vi "Create Table.vi"(8 "error in (no error)":errorcluster, 9 "New Table Name":string, 10 "Table Paths":string[](array[string]), 11 "Data.PGSQL":refnum<class "LV-Data.PGSQL.lvclass">) -> (0 "error out":errorcluster, 3 "Data.PGSQL out":refnum<class "LV-Data.PGSQL.lvclass">)   [LabVIEW 2019, in "LV-Data.PGSQL.lvclass"]
uses:
  LV-Data.PGSQL.lvclass
panel:
  in  "OK":bool
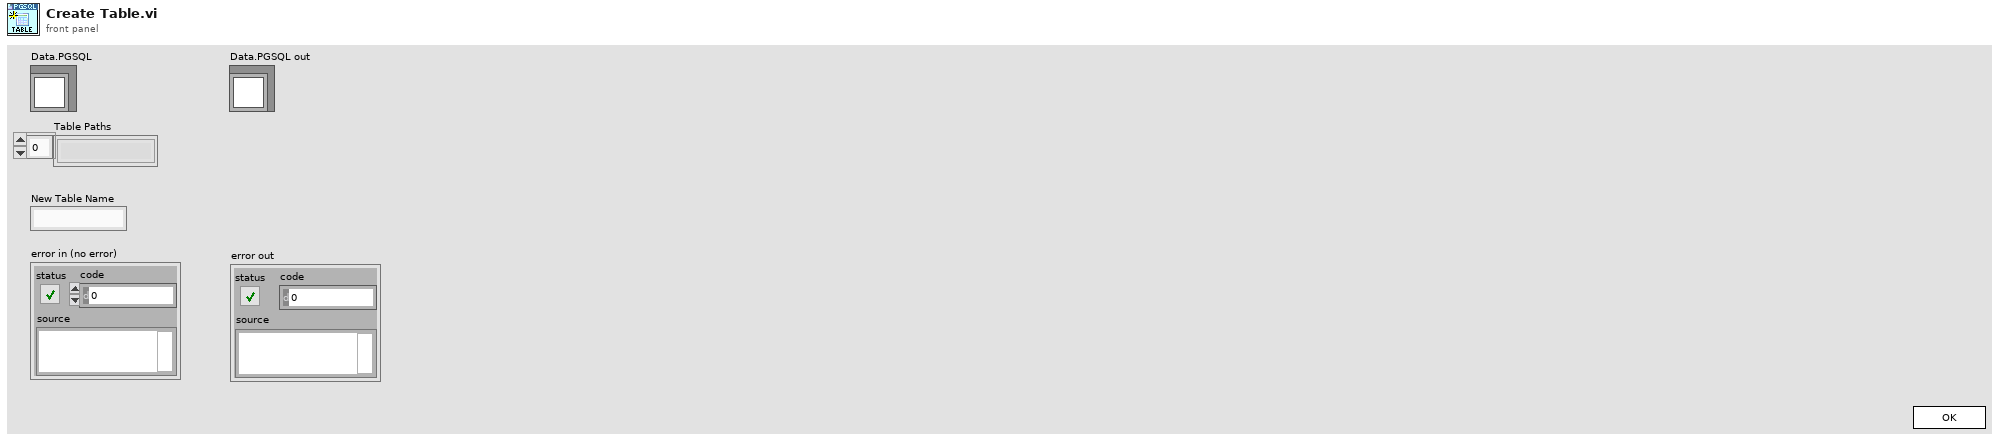
[diagram p1: front panel]
types:
  T1 = enum32{"Invalid", "Standard", "Closed", "Hidden", "Minimized", "Maximized"}
  T2 = enum32{"invalid app kind", "Development System", "Run Time System", "Student Edition", "Embedded LabVIEW", "Evaluation", "Custom"}
  T3 = cluster{"Core":cluster{"Current VI Reference":refnum<vi>, "Close Panel on Exit?":bool}, "LV-Data.PGSQL out":refnum<class "LV-Data.PGSQL.lvclass">, "Table Paths":string[], "New Table Name":string, "New Table Number":string}
  T4 = cluster{"Current VI Reference":refnum<vi>, "Close Panel on Exit?":bool}
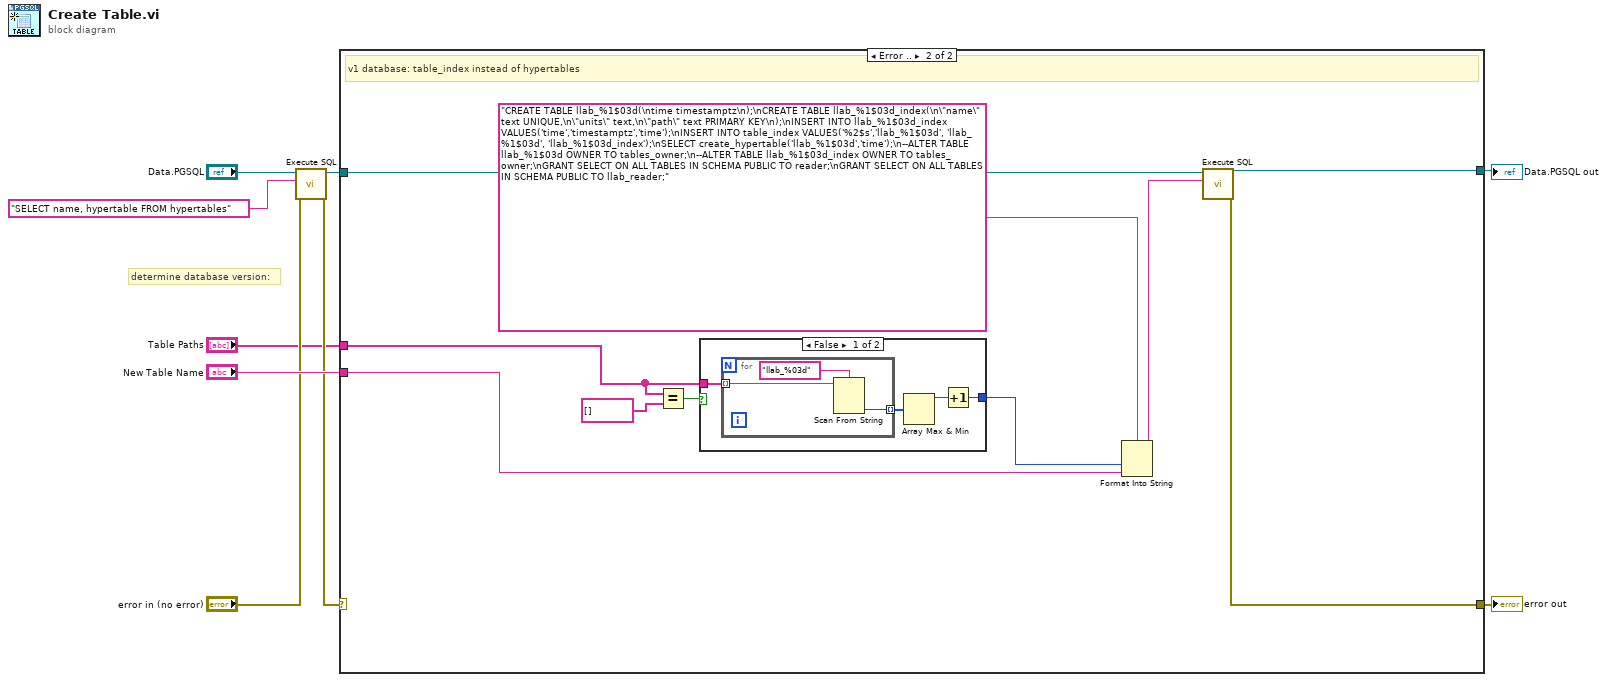
[diagram p0: block diagram]
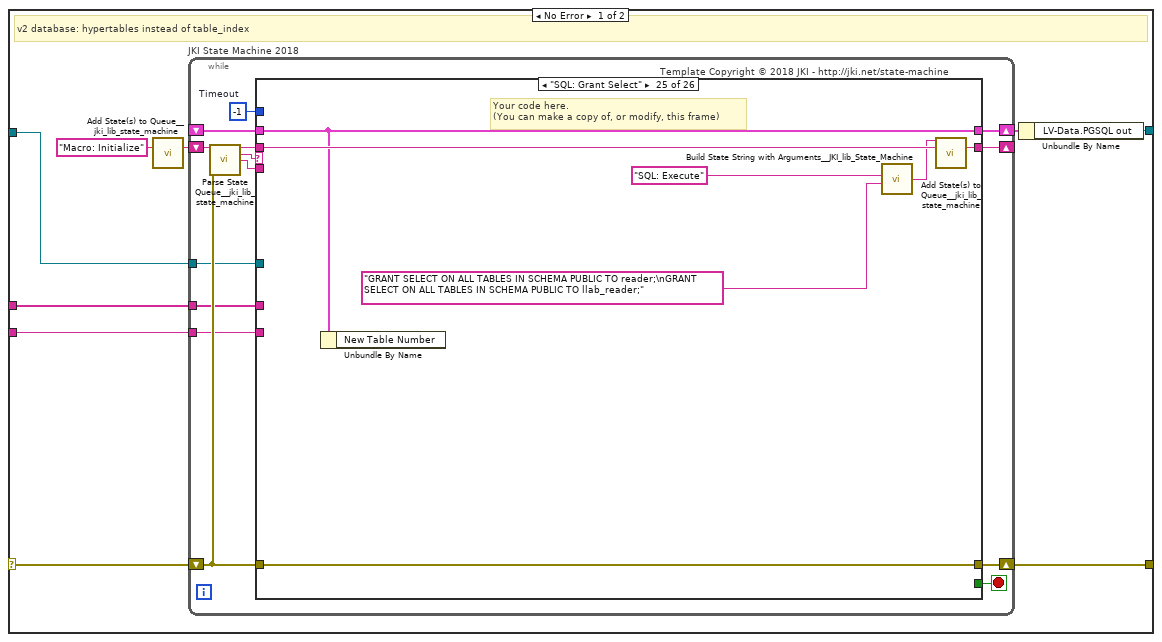
[diagram p2: hidden frame]
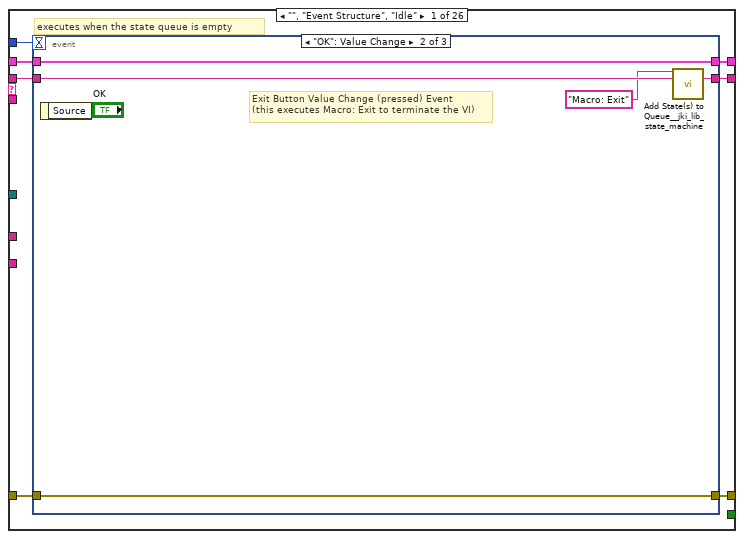
[diagram p3: hidden frame]
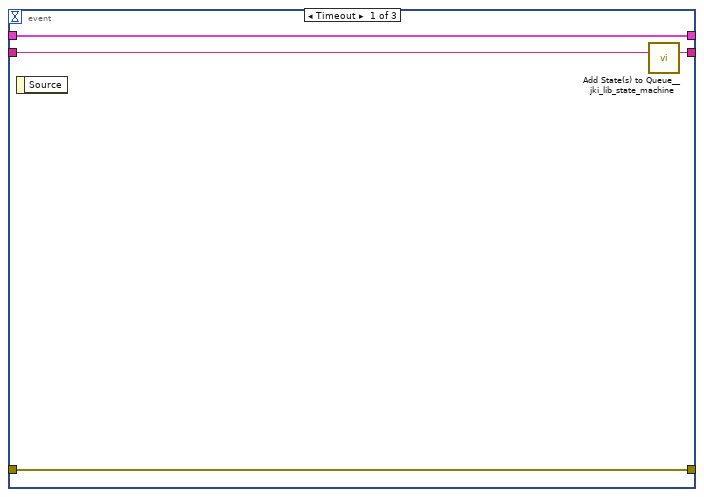
[diagram p4: hidden frame]
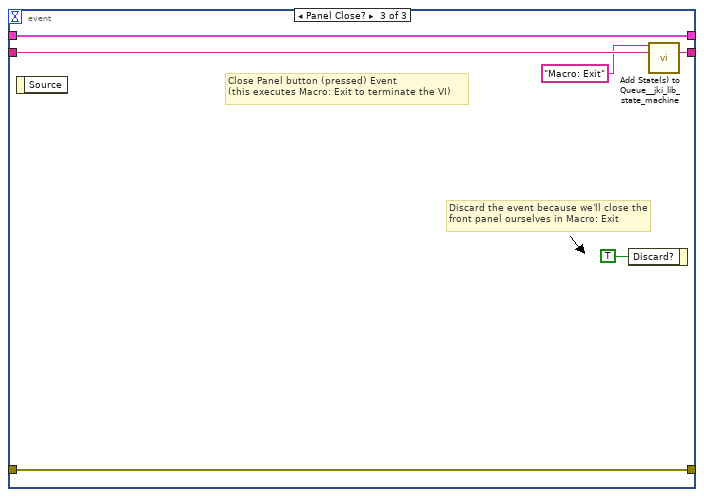
[diagram p5: hidden frame]
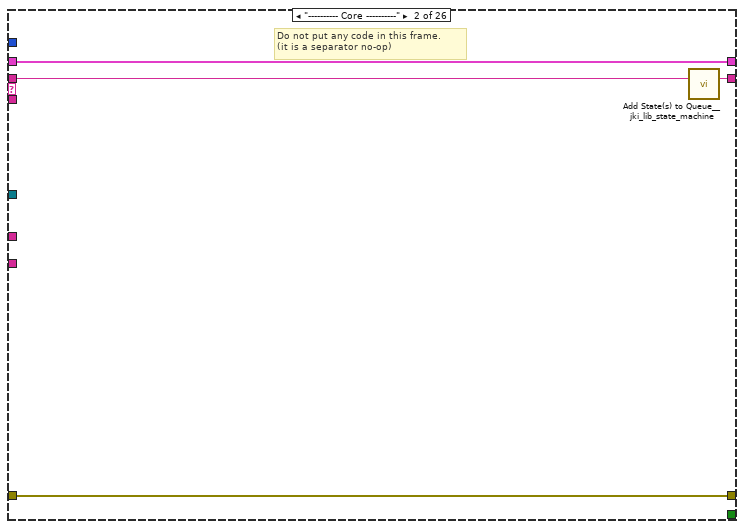
[diagram p6: hidden frame]
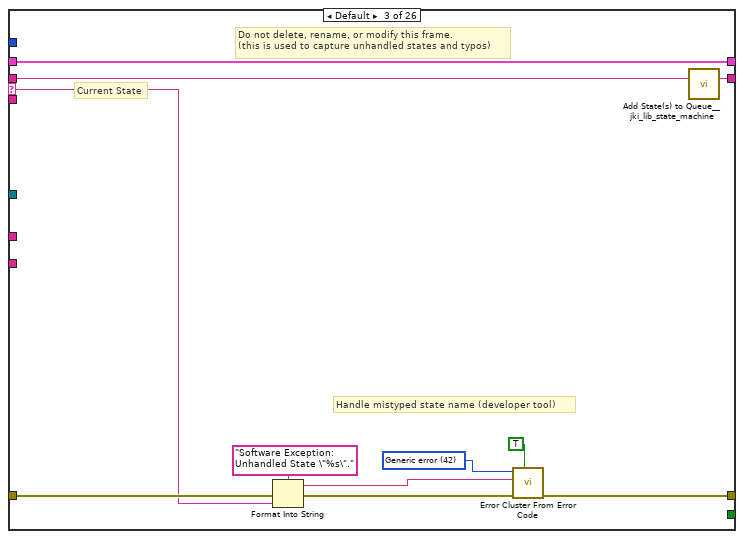
[diagram p7: hidden frame]
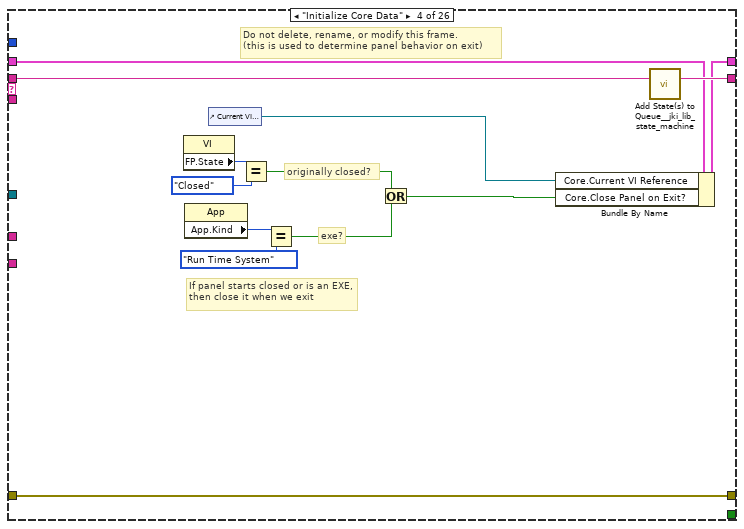
[diagram p8: hidden frame]
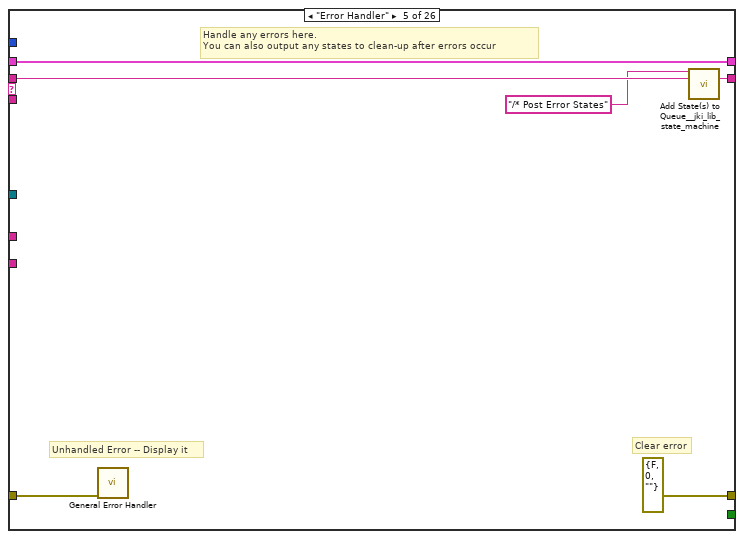
[diagram p9: hidden frame]
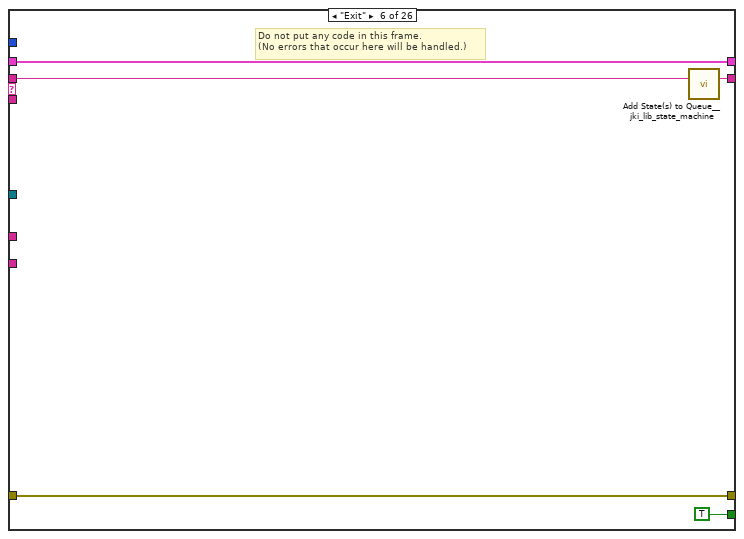
[diagram p10: hidden frame]
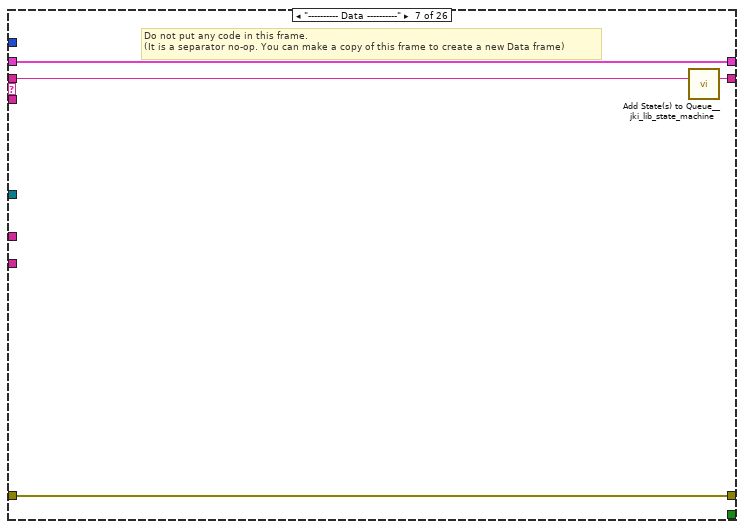
[diagram p11: hidden frame]
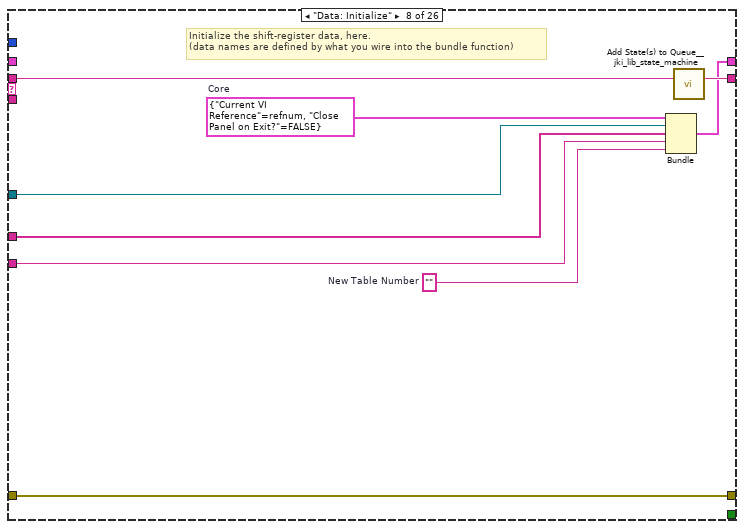
[diagram p12: hidden frame]
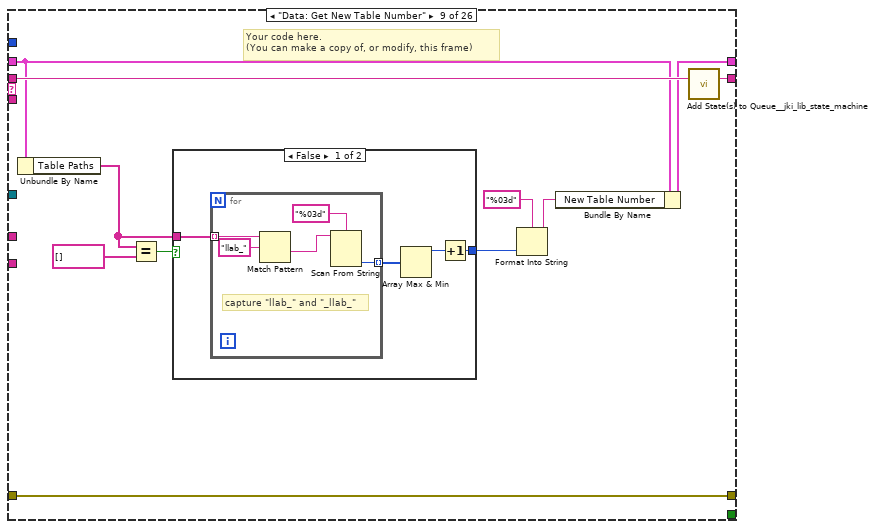
[diagram p13: hidden frame]
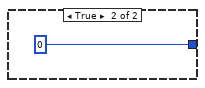
[diagram p14: hidden frame]
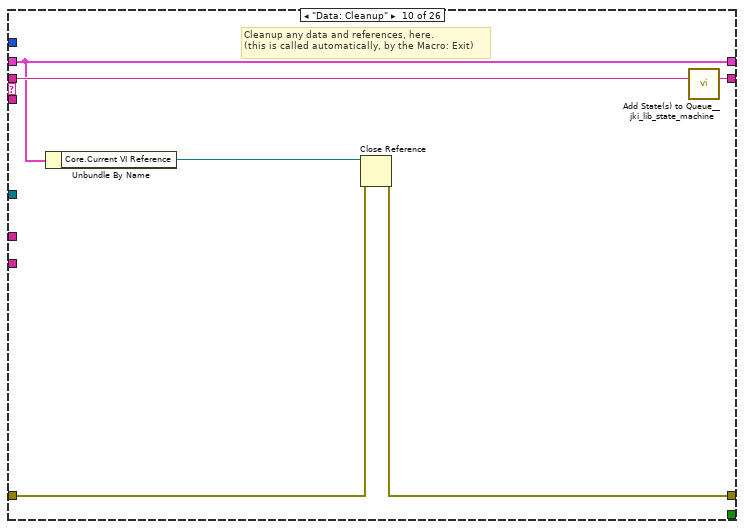
[diagram p15: hidden frame]
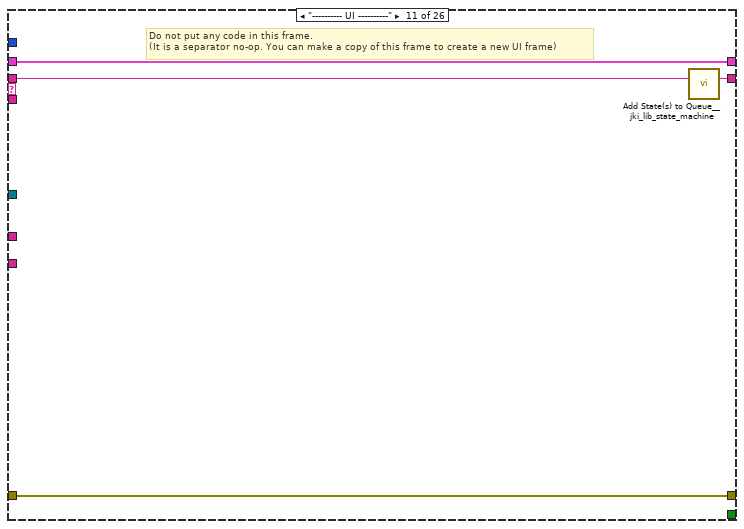
[diagram p16: hidden frame]
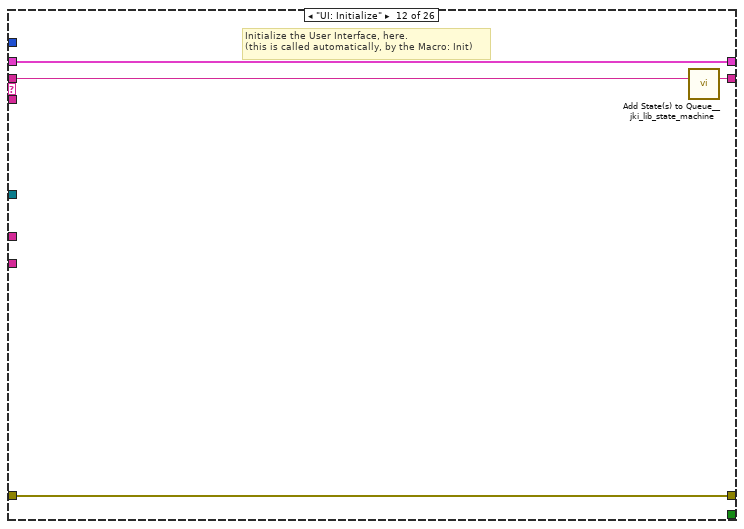
[diagram p17: hidden frame]
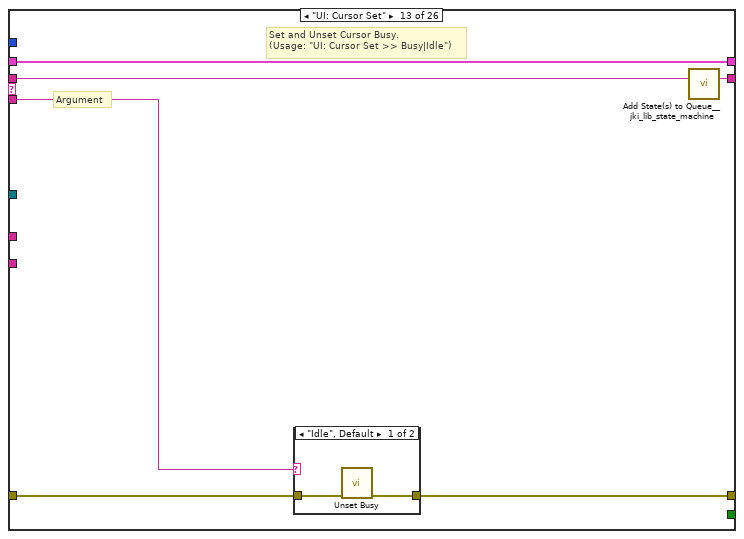
[diagram p18: hidden frame]
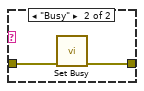
[diagram p19: hidden frame]
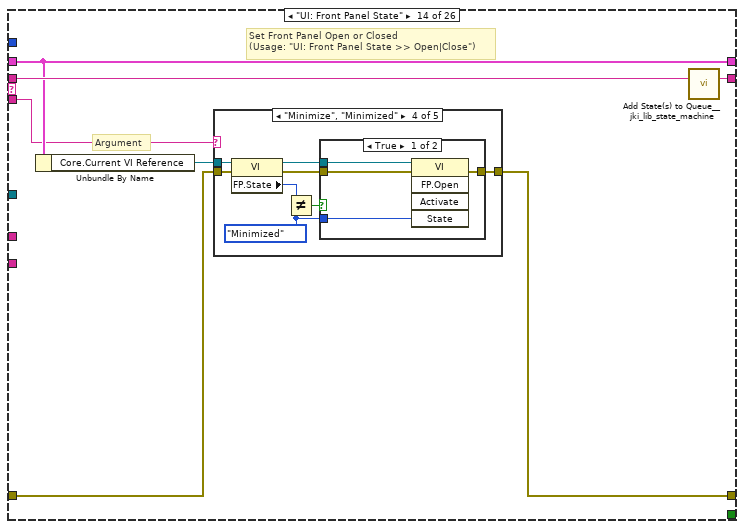
[diagram p20: hidden frame]
diagram:
  # "determine database version:"
  n1 = call "Execute SQL.vi"("error in"="error in (no error)", "SQL"="SELECT name, hypertable FROM hypertables" ("command"), "LV-Data.PGSQL"="Data.PGSQL") -> ("error out"=w5:errorcluster, "LV-Data.PGSQL out"=w3:refnum<class "LV-Data.PGSQL.lvclass">)  [unwired: 5 in, 2 out]
  n2 = case shown="Error .." w5 {
    selector: w5 -> [w15 _]
    tunnel: [w18 w318] -> w9
    tunnel: [w17 w319] -> w8
    tunnel: "New Table Name" -> [w16 w314]
    tunnel: w3 -> [w11 w317]
    tunnel: "Table Paths" -> [w10 w316]
    frame No Error {
      # "v2 database: hypertables instead of table_index"
      n3 = call <vilib>:"Add State(s) to Queue__jki_lib_state_machine.vi"("State(s) in (\"\")"="Macro: Initialize") -> ("States Out"=w14:string)  [unwired: 14 in]
      n4 = while "JKI State Machine 2018" {
        shift-right: [w25] -> w12
        shift-left: _ -> [w24]
        shift-right: [w28] -> w17
        shift-left: w15 -> [w22]
        shift-right: [w27] -> _
        shift-left: w14 -> [w29]
        tunnel: w11 -> [w21]
        tunnel: w16 -> [w20]
        tunnel: w10 -> [w19]
        stop <- w26 stop-if-true
        w23 = -1  # Timeout
        # "Template Copyright © 2018 JKI - http://jki.net/state-machine"
        n5 = call <vilib>:"Parse State Queue__jki_lib_state_machine.vi"("State Queue"=w29, "Error In (no error)"=w22) -> ("Remaining States"=w31:string, "Current State"=w32:string, "Arguments"=w30:string)  [unwired: 11 in]
        n6 = case shown="\"SQL: Grant Select\"" w32 {
          selector: w32 -> [_ _ w59 _ _ _ _ _ _ _ _ _ _ _ _ _ _ _ _ _ _ _ _ _ _ _]
          tunnel: w31 -> [w39 w58 w63 w82 w88 w93 w97 w106 w117 w133 w137 w141 w147 w158 w227 w232 w237 w247 w251 w260 w269 w278 w288 w297 w304 w313]
          tunnel: w30 -> [_ _ _ _ _ _ _ _ _ _ _ _ w142 w152 _ _ _ _ _ _ _ _ _ _ _ w308]
          tunnel: w24 -> [w37 w55 w61 w75 w85 w91 w94 _ w109 w128 w134 w139 w145 w154 w224 w229 w234 w244 w248 w257 w266 w275 w285 w294 w301 w305]
          tunnel: [w36 w56 w65 w79 errorcluster {"status"=FALSE, "code"=0, "source"=""} ("error out") w90 w95 w103 w115 w129 w135 w138 w143 w155 w225 w230 w235 w245 w249 w258 w267 w276 w286 w295 w302 w310] -> w28
          tunnel: w22 -> [w35 w56 w64 w79 w84 w90 w95 w103 w115 w130 w135 w138 w144 w156 w225 w230 w235 w245 w249 w258 w267 w276 w286 w295 w302 w309]
          tunnel: [w38 w57 w62 w81 w87 w92 w96 w105 w116 w132 w136 w140 w146 w157 w226 w231 w236 w246 w250 w259 w268 w277 w287 w296 w303 w312] -> w27
          tunnel: [_ _ _ _ _ TRUE _ _ _ _ _ _ _ _ _ _ _ _ _ _ _ _ _ _ _ _] -> w26
          tunnel: [w34 w55 w61 w80 w85 w91 w94 w104 w111 w128 w134 w139 w145 w154 w224 w229 w234 w244 w248 w257 w266 w275 w285 w294 w301 w306] -> w25
          tunnel: w23 -> [w33 _ _ _ _ _ _ _ _ _ _ _ _ _ _ _ _ _ _ _ _ _ _ _ _ _]
          tunnel: w21 -> [_ _ _ _ _ _ _ w99 _ _ _ _ _ _ _ _ _ _ _ _ _ _ _ _ _ _]
          tunnel: w20 -> [_ _ _ _ _ _ _ w100 _ _ _ _ _ _ _ _ _ _ _ _ _ _ _ _ _ _]
          tunnel: w19 -> [_ _ _ _ _ _ _ w98 _ _ _ _ _ _ _ _ _ _ _ _ _ _ _ _ _ _]
          frame "", "Event Structure", "Idle" {
            # "executes when the state queue is empty"
            n7 = event shown="[1] \"OK\": Value Change" {
              selector: _ -> [_ _ _]
              dyn-events: _ -> [_ _ _]
              timeout: w33 -> [_ _ _]
              tunnel: w39 -> [w43 w48 w54]
              tunnel: [w42 w47 w53] -> w38
              tunnel: w37 -> [w40 w45 w51]
              tunnel: [w41 w46 w52] -> w36
              tunnel: w35 -> [w41 w46 w52]
              tunnel: [w40 w45 w51] -> w34
              event Timeout {
                n8 = event-data() -> ()  [unwired: 1 in, 1 out]
                n9 = call <vilib>:"Add State(s) to Queue__jki_lib_state_machine.vi"("State(s) in (\"\")"=w43) -> ("States Out"=w42:string)  [unwired: 14 in]
              }
              event "OK": Value Change {
                # "Exit Button Value Change (pressed) Event\n(this executes Macro: Exit to terminate the VI)"
                n10 = event-data() -> ()  [unwired: 1 in, 1 out]
                n11 = call <vilib>:"Add State(s) to Queue__jki_lib_state_machine.vi"("State(s) in Front (\"\")"="Macro: Exit", "State(s) in (\"\")"=w48) -> ("States Out"=w47:string)  [unwired: 13 in]
              }
              event Panel Close? {
                # "Discard the event because we'll close the front panel ourselves in Macro: Exit"
                # "Close Panel button (pressed) Event\n(this executes Macro: Exit to terminate the VI)"
                n12 = event-data() -> ()  [unwired: 1 in, 1 out]
                n13 = event-data("Discard?"=TRUE) -> ()  [unwired: 1 in, 1 out]
                n14 = call <vilib>:"Add State(s) to Queue__jki_lib_state_machine.vi"("State(s) in Front (\"\")"="Macro: Exit", "State(s) in (\"\")"=w54) -> ("States Out"=w53:string)  [unwired: 13 in]
              }
            }
          }
          frame "---------- Core ----------" {
            # "Do not put any code in this frame.\n(it is a separator no-op)"
            n15 = call <vilib>:"Add State(s) to Queue__jki_lib_state_machine.vi"("State(s) in (\"\")"=w58) -> ("States Out"=w57:string)  [unwired: 14 in]
          }
          frame Default {
            w68 = 42 items=["No error", "Argument error", "Memory is full", "Out of zone", "End of file", "File already open", "Generic file I/O error", "File not found", "File permission error", "Disk is full", "Duplicate path", "Too many files open", "System feature not enabled", "Resource file not found", "Cannot add resource", "Resource not found", "Image not found", "Image memory error", "Pen does not exist", "Config type invalid", "Config token not found", "Config parse error", "Config memory error", "Bad external code format", "Bad external code offset", "External code not present", "Null window", "Destroy window error", "Null menu", "Print aborted", "Bad print record", "Print driver error", "Windows error during printing", "Memory error during printing", "Print dialog error", "Generic print error", "Invalid device refnum", "Device not found", "Device parameter error", "Device unit error", "Cannot open device", "Device call aborted", "Generic error", "Cancelled by user", "Object ID too low", "Object ID too high", "Object not in heap", "Unknown heap", "Unknown object (invalid DefProc)", "Unknown object (DefProc not in table)", "Message out of range", "Invalid (null) method", "Unknown message", "Manager call not supported", "Bad address", "Network operation in progress", "Network operation timed out", "Connection is busy", "Network attribute not supported", "Network error", "Address in use", "System out of memory", "Connection aborted", "Connection refused", "Not connected", "Already connected", "Connection closed", "Initialization error (interapplication manager)", "Bad occurrence", "Wait on unbound occurrence handler", "Occurrence queue overflow", "Datalog type conflict", "Unused", "Unrecognized type (interapplication manager)", "Memory corrupt", "Failed to make temporary DLL", "Old CIN version", "Drag socket not found", "Failed to load drop-object", "Failed to register OLE object", "Failed to release OLE object", "Format specifier type mismatch", "Unknown format specifier", "Too few format specifiers", "Too many format specifiers", "Scan failed", "Newer CIN version", "Error converting to variant", "Runtime menu error", "Password tampered", "Variant attribute not found", "Incompatible variant data type", "Event data is not available", "Event Store is not present", "Occurrence is not found", "Event Queue is not created", "Event info is not available", "Refnum passed is NULL", "Error retrieving Class GUID", "Error retrieving CoClass GUID", "Error retrieving TypeLib GUID.", "Bad built application magic bytes.", "Specific driver is different from the specific driver associated with the Logical Name.", "There is no session opened to the class driver.", "Max Error", "MAX - Error with config objects", "MAX - Error loading configuration", "MAX - Group not supported"]
            # "Current State"
            # "Do not delete, rename, or modify this frame.\n(this is used to capture unhandled states and typos)"
            # "Handle mistyped state name (developer tool)"
            n16 = Format Into String(format string="Software Exception: Unhandled State \"%s\"." ("message"), error in=w64, w59) -> (resulting string=w67:string, error out=w66:errorcluster)  [unwired: 1 in]
            n17 = call <vilib>:"Error Cluster From Error Code.vi"("show call chain? (False)"=TRUE, "error in (no error)"=w66, "error message (\"\")"=w67, "error code (0)"=w68) -> ("error out"=w65:errorcluster)  [unwired: 5 in]
            n18 = call <vilib>:"Add State(s) to Queue__jki_lib_state_machine.vi"("State(s) in (\"\")"=w63) -> ("States Out"=w62:string)  [unwired: 14 in]
          }
          frame "Initialize Core Data" {
            # "Do not delete, rename, or modify this frame.\n(this is used to determine panel behavior on exit)"
            # "originally closed?"
            # "exe?"
            # "If panel starts closed or is an EXE, then close it when we exit"
            n19 = property class="VI"() -> ("FP.State"=w72:T1)  [unwired: 2 in, 2 out]
            n20 = property class="App"() -> ("App.Kind"=w78:T2)  [unwired: 2 in, 2 out]
            n21 = control-ref of="Current VI Reference"() -> (w73:refnum<vi>)
            n22 = Equal?(x=w72, y=T1."Closed" ("Front Panel Window:State")) -> (x = y?=w70:bool)
            n23 = Equal?(x=w78, y=T2."Run Time System" ("Application:Kind")) -> (x = y?=w76:bool)
            n24 = Or(x=w70, y=w76) -> (x .or. y?=w74:bool)
            n25 = Bundle By Name(cluster=w75, "Core.Current VI Reference"=w73, "Core.Close Panel on Exit?"=w74) -> (w80:T3)
            n26 = call <vilib>:"Add State(s) to Queue__jki_lib_state_machine.vi"("State(s) in (\"\")"=w82) -> ("States Out"=w81:string)  [unwired: 14 in]
          }
          frame "Error Handler" {
            # "Unhandled Error -- Display it"
            # "Handle any errors here.\nYou can also output any states to clean-up after errors occur"
            # "Clear error"
            n27 = call <vilib>:"General Error Handler.vi"("error in (no error)"=w84) -> ()  [unwired: 10 in, 5 out]
            n28 = call <vilib>:"Add State(s) to Queue__jki_lib_state_machine.vi"("State(s) in Front (\"\")"="/* Post Error States", "State(s) in (\"\")"=w88) -> ("States Out"=w87:string)  [unwired: 13 in]
          }
          frame "Exit" {
            # "Do not put any code in this frame.\n(No errors that occur here will be handled.)"
            n29 = call <vilib>:"Add State(s) to Queue__jki_lib_state_machine.vi"("State(s) in (\"\")"=w93) -> ("States Out"=w92:string)  [unwired: 14 in]
          }
          frame "---------- Data ----------" {
            # "Do not put any code in this frame.\n(It is a separator no-op. You can make a copy of this frame to create a new Data frame)"
            n30 = call <vilib>:"Add State(s) to Queue__jki_lib_state_machine.vi"("State(s) in (\"\")"=w97) -> ("States Out"=w96:string)  [unwired: 14 in]
          }
          frame "Data: Initialize" {
            w101 = ""  # New Table Number
            w102 = T4 {"Current VI Reference"=refnum, "Close Panel on Exit?"=FALSE}  # Core
            # "Initialize the shift-register data, here.\n(data names are defined by what you wire into the bundle function)"
            n31 = Bundle("Core"=w102, "LV-Data.PGSQL out"=w99, "Table Paths"=w98, "New Table Name"=w100, "New Table Number"=w101) -> (w104:T3)  [unwired: 1 in]
            n32 = call <vilib>:"Add State(s) to Queue__jki_lib_state_machine.vi"("State(s) in (\"\")"=w106) -> ("States Out"=w105:string)  [unwired: 14 in]
          }
          frame "Data: Get New Table Number" {
            # "Your code here.\n(You can make a copy of, or modify, this frame)"
            n33 = Unbundle By Name(w109) -> ("Table Paths"=w108:string[])
            n34 = Equal?(x=w108, y=string[] []) -> (x = y?=w110:bool)
            n35 = case shown="False" w110 {
              tunnel: w108 -> [w121 _]
              tunnel: [w118 0] -> w113
              frame False {
                n36 = for {
                  tunnel: w121 -> [w124] mode=indexing
                  tunnel: [w125] -> w120 mode=indexing
                  # "capture \"llab_\" and \"_llab_\""
                  n37 = Match Pattern(string=w124, regular expression="llab_") -> (after substring=w122:string)  [unwired: 1 in, 3 out]
                  n38 = Scan From String(format string="%03d", input string=w122) -> (output 1=w125:i32)  [unwired: 3 in, 3 out]
                }
                n39 = Array Max & Min(array=w120) -> (max value=w119:i32)  [unwired: 3 out]
                n40 = Increment(x=w119) -> (x+1=w118:i32)
              }
              frame True {
              }
            }
            n41 = Format Into String(format string="%03d", w113) -> (resulting string=w107:string)  [unwired: 2 in, 1 out]
            n42 = Bundle By Name(cluster=w109, "New Table Number"=w107) -> (w111:T3)
            n43 = call <vilib>:"Add State(s) to Queue__jki_lib_state_machine.vi"("State(s) in (\"\")"=w117) -> ("States Out"=w116:string)  [unwired: 14 in]
          }
          frame "Data: Cleanup" {
            # "Cleanup any data and references, here.\n(this is called automatically, by the Macro: Exit)"
            n44 = Unbundle By Name(w128) -> ("Core.Current VI Reference"=w131:refnum<vi>)
            n45 = Close Reference(reference=w131, error in (no error)=w130) -> (error out=w129:errorcluster)
            n46 = call <vilib>:"Add State(s) to Queue__jki_lib_state_machine.vi"("State(s) in (\"\")"=w133) -> ("States Out"=w132:string)  [unwired: 14 in]
          }
          frame "---------- UI ----------" {
            # "Do not put any code in this frame.\n(It is a separator no-op. You can make a copy of this frame to create a new UI frame)"
            n47 = call <vilib>:"Add State(s) to Queue__jki_lib_state_machine.vi"("State(s) in (\"\")"=w137) -> ("States Out"=w136:string)  [unwired: 14 in]
          }
          frame "UI: Initialize" {
            # "Initialize the User Interface, here.\n(this is called automatically, by the Macro: Init)"
            n48 = call <vilib>:"Add State(s) to Queue__jki_lib_state_machine.vi"("State(s) in (\"\")"=w141) -> ("States Out"=w140:string)  [unwired: 14 in]
          }
          frame "UI: Cursor Set" {
            # "Argument"
            # "Set and Unset Cursor Busy.\n(Usage: \"UI: Cursor Set >> Busy|Idle\")"
            n49 = case shown="\"Idle\", Default" w142 {
              tunnel: w144 -> [w149 w151]
              tunnel: [w148 w150] -> w143
              frame "Idle", Default {
                n50 = call <vilib>:"Unset Busy.vi"("error in (no error)"=w149) -> ("error out"=w148:errorcluster)  [unwired: 10 in]
              }
              frame "Busy" {
                n51 = call <vilib>:"Set Busy.vi"("error in (no error)"=w151) -> ("error out"=w150:errorcluster)  [unwired: 9 in, 1 out]
              }
            }
            n52 = call <vilib>:"Add State(s) to Queue__jki_lib_state_machine.vi"("State(s) in (\"\")"=w147) -> ("States Out"=w146:string)  [unwired: 14 in]
          }
          frame "UI: Front Panel State" {
            # "Argument"
            # "Set Front Panel Open or Closed\n(Usage: \"UI: Front Panel State >> Open|Close\")"
            n53 = Unbundle By Name(w154) -> ("Core.Current VI Reference"=w153:refnum<vi>)
            n54 = case shown="\"Minimize\", \"Minimized\"" w152 {
              tunnel: w156 -> [w164 w179 w190 w203 w216]
              tunnel: [w166 w180 w192 w205 w218] -> w155
              tunnel: w153 -> [w165 w177 w191 w204 w217]
              frame "Open", "Standard", Default {
                w159 = T1."Standard" ("State")
                n55 = property class="VI"(reference=w165, error in=w164) -> (reference out=w162:refnum<vi>, error out=w163:errorcluster, "FP.State"=w161:T1)
                n56 = Not Equal?(x=w161, y=w159) -> (x != y?=w160:bool)
                n57 = case shown="True" w160 {
                  tunnel: [w170 w172] -> w166
                  tunnel: w163 -> [w169 w172]
                  tunnel: w162 -> [w168 _]
                  tunnel: w159 -> [w167 _]
                  frame True {
                    n58 = invoke class="VI" method="FP.Open"(reference=w168, error in=w169, "Activate"=TRUE, "State"=w167) -> (error out=w170:errorcluster)  [unwired: 1 in, 4 out]
                  }
                  frame False {
                  }
                }
              }
              frame "Close", "Closed" {
                n59 = property class="VI"(reference=w177, error in=w179) -> (reference out=w176:refnum<vi>, error out=w178:errorcluster, "FP.State"=w174:T1)
                n60 = Not Equal?(x=w174, y=T1."Closed" ("Front Panel Window:State")) -> (x != y?=w173:bool)
                n61 = case shown="True" w173 {
                  tunnel: [w181 w184] -> w180
                  tunnel: w178 -> [w181 w183]
                  tunnel: w176 -> [_ w182]
                  frame False {
                  }
                  frame True {
                    n62 = invoke class="VI" method="FP.Close"(reference=w182, error in=w183) -> (error out=w184:errorcluster)  [unwired: 1 in, 2 out]
                  }
                }
              }
              frame "Hidden", "Hide" {
                w185 = T1."Hidden" ("State")
                n63 = property class="VI"(reference=w191, error in=w190) -> (reference out=w188:refnum<vi>, error out=w189:errorcluster, "FP.State"=w187:T1)
                n64 = Not Equal?(x=w187, y=w185) -> (x != y?=w186:bool)
                n65 = case shown="True" w186 {
                  tunnel: [w196 w197] -> w192
                  tunnel: w189 -> [w195 w197]
                  tunnel: w188 -> [w194 _]
                  tunnel: w185 -> [w193 _]
                  frame True {
                    n66 = invoke class="VI" method="FP.Open"(reference=w194, error in=w195, "State"=w193) -> (error out=w196:errorcluster)  [unwired: 2 in, 4 out]
                  }
                  frame False {
                  }
                }
              }
              frame "Minimize", "Minimized" {
                w198 = T1."Minimized" ("State")
                n67 = property class="VI"(reference=w204, error in=w203) -> (reference out=w201:refnum<vi>, error out=w202:errorcluster, "FP.State"=w200:T1)
                n68 = Not Equal?(x=w200, y=w198) -> (x != y?=w199:bool)
                n69 = case shown="True" w199 {
                  tunnel: [w209 w210] -> w205
                  tunnel: w202 -> [w208 w210]
                  tunnel: w201 -> [w207 _]
                  tunnel: w198 -> [w206 _]
                  frame True {
                    n70 = invoke class="VI" method="FP.Open"(reference=w207, error in=w208, "State"=w206) -> (error out=w209:errorcluster)  [unwired: 2 in, 4 out]
                  }
                  frame False {
                  }
                }
              }
              frame "Maximize", "Maximized" {
                w211 = T1."Maximized" ("State")
                n71 = property class="VI"(reference=w217, error in=w216) -> (reference out=w214:refnum<vi>, error out=w215:errorcluster, "FP.State"=w213:T1)
                n72 = Not Equal?(x=w213, y=w211) -> (x != y?=w212:bool)
                n73 = case shown="True" w212 {
                  tunnel: [w222 w223] -> w218
                  tunnel: w215 -> [w221 w223]
                  tunnel: w214 -> [w220 _]
                  tunnel: w211 -> [w219 _]
                  frame True {
                    n74 = invoke class="VI" method="FP.Open"(reference=w220, error in=w221, "State"=w219) -> (error out=w222:errorcluster)  [unwired: 2 in, 4 out]
                  }
                  frame False {
                  }
                }
              }
            }
            n75 = call <vilib>:"Add State(s) to Queue__jki_lib_state_machine.vi"("State(s) in (\"\")"=w158) -> ("States Out"=w157:string)  [unwired: 14 in]
          }
          frame "---------- Macro ----------" {
            # "Do not put any code in this frame.\n(It is a separator no-op. You can make a copy of this frame to create a new Macro frame)"
            n76 = call <vilib>:"Add State(s) to Queue__jki_lib_state_machine.vi"("State(s) in (\"\")"=w227) -> ("States Out"=w226:string)  [unwired: 14 in]
          }
          frame "Macro: Initialize" {
            w228 = "Data: Initialize\nInitialize Core Data\nUI: Initialize\nUI: Front Panel State >> Close\nMacro: Create Table\nMacro: Exit"  # Data: Initialize Initialize Core Data UI: Initialize UI: Front Panel State >> Close Macro: Create Table Macro: Exit
            # "Initialization Macro\n(This is called once, when the VI starts)"
            n77 = call <vilib>:"Add State(s) to Queue__jki_lib_state_machine.vi"("State(s) in Front (\"\")"=w228, "State(s) in (\"\")"=w232) -> ("States Out"=w231:string)  [unwired: 13 in]
          }
          frame "Macro: Create Table" {
            # "Do not put any code in this frame.\n(It is a separator no-op. You can make a copy of this frame to create a new Macro frame)"
            n78 = call <vilib>:"Add State(s) to Queue__jki_lib_state_machine.vi"("State(s) in Front (\"\")"="SQL: Create Table\nSQL: Create Index Table\nSQL: Insert Into Index Table\nSQL: Insert Into Hypertables\nSQL: Create Hypertable\nSQL: Grant Select" ("State(s) in Front (\"\")"), "State(s) in (\"\")"=w237) -> ("States Out"=w236:string)  [unwired: 13 in]
          }
          frame "Macro: Exit" {
            # "Exit Macro\n(This is called once, when the VI exits)"
            n79 = Unbundle By Name(w244) -> ("Core.Close Panel on Exit?"=w243:bool)
            n80 = Select(t="UI: Front Panel State >> Close", s=w243, f="") -> (s? t:f=w240:string)
            n81 = call <vilib>:"Add State(s) to Queue__jki_lib_state_machine.vi"("State(s) in (\"\")"=w240, "State(s) at Back (\"\")"="Data: Cleanup\nExit") -> ("States Out"=w238:string)  [unwired: 13 in]
            n82 = call <vilib>:"Add State(s) to Queue__jki_lib_state_machine.vi"("State(s) in Front (\"\")"=w238, "State(s) in (\"\")"=w247) -> ("States Out"=w246:string)  [unwired: 13 in]
          }
          frame "---------- SQL ----------" {
            # "Template Separator\n(You can make a copy of, or modify, this frame)"
            n83 = call <vilib>:"Add State(s) to Queue__jki_lib_state_machine.vi"("State(s) in (\"\")"=w251) -> ("States Out"=w250:string)  [unwired: 14 in]
          }
          frame "SQL: Create Table" {
            # "Your code here.\n(You can make a copy of, or modify, this frame)"
            n84 = Unbundle By Name(w257) -> ("New Table Number"=w255:string)
            n85 = Format Into String(format string="CREATE TABLE _llab_%s (time timestamptz);", w255) -> (resulting string=w252:string)  [unwired: 2 in, 1 out]
            n86 = call <vilib>:"Build State String with Arguments__JKI_lib_State_Machine.vi"("Arguments (\"\")"=w252, "State"="SQL: Execute") -> ("State with Arguments"=w253:string)  [unwired: 4 in]
            n87 = call <vilib>:"Add State(s) to Queue__jki_lib_state_machine.vi"("State(s) in Front (\"\")"=w253, "State(s) in (\"\")"=w260) -> ("States Out"=w259:string)  [unwired: 13 in]
          }
          frame "SQL: Create Index Table" {
            # "Your code here.\n(You can make a copy of, or modify, this frame)"
            n88 = Unbundle By Name(w266) -> ("New Table Number"=w264:string)
            n89 = Format Into String(format string="CREATE TABLE _llab_%s_index(\n\"name\" text UNIQUE,\n\"units\" text,\n\"path\" text PRIMARY KEY\n);", w264) -> (resulting string=w261:string)  [unwired: 2 in, 1 out]
            n90 = call <vilib>:"Build State String with Arguments__JKI_lib_State_Machine.vi"("Arguments (\"\")"=w261, "State"="SQL: Execute") -> ("State with Arguments"=w262:string)  [unwired: 4 in]
            n91 = call <vilib>:"Add State(s) to Queue__jki_lib_state_machine.vi"("State(s) in Front (\"\")"=w262, "State(s) in (\"\")"=w269) -> ("States Out"=w268:string)  [unwired: 13 in]
          }
          frame "SQL: Insert Into Index Table" {
            # "Your code here.\n(You can make a copy of, or modify, this frame)"
            n92 = Unbundle By Name(w275) -> ("New Table Number"=w273:string)
            n93 = Format Into String(format string="INSERT INTO _llab_%s_index VALUES('time','timestamptz','time');", w273) -> (resulting string=w270:string)  [unwired: 2 in, 1 out]
            n94 = call <vilib>:"Build State String with Arguments__JKI_lib_State_Machine.vi"("Arguments (\"\")"=w270, "State"="SQL: Execute") -> ("State with Arguments"=w271:string)  [unwired: 4 in]
            n95 = call <vilib>:"Add State(s) to Queue__jki_lib_state_machine.vi"("State(s) in Front (\"\")"=w271, "State(s) in (\"\")"=w278) -> ("States Out"=w277:string)  [unwired: 13 in]
          }
          frame "SQL: Insert Into Hypertables" {
            # "Your code here.\n(You can make a copy of, or modify, this frame)"
            n96 = Unbundle By Name(w285) -> ("New Table Name"=w279:string, "New Table Number"=w283:string)
            n97 = Format Into String(format string="INSERT INTO hypertables\n(\"name\", hypertable, hypertable_index)\nVALUES('%1$s','_llab_%2$s', '_llab_%2$s_index');", w279, w283) -> (resulting string=w280:string)  [unwired: 2 in, 1 out]
            n98 = call <vilib>:"Build State String with Arguments__JKI_lib_State_Machine.vi"("Arguments (\"\")"=w280, "State"="SQL: Execute") -> ("State with Arguments"=w281:string)  [unwired: 4 in]
            n99 = call <vilib>:"Add State(s) to Queue__jki_lib_state_machine.vi"("State(s) in Front (\"\")"=w281, "State(s) in (\"\")"=w288) -> ("States Out"=w287:string)  [unwired: 13 in]
          }
          frame "SQL: Create Hypertable" {
            # "Your code here.\n(You can make a copy of, or modify, this frame)"
            n100 = Unbundle By Name(w294) -> ("New Table Number"=w292:string)
            n101 = Format Into String(format string="SELECT create_hypertable('_llab_%s','time');", w292) -> (resulting string=w289:string)  [unwired: 2 in, 1 out]
            n102 = call <vilib>:"Build State String with Arguments__JKI_lib_State_Machine.vi"("Arguments (\"\")"=w289, "State"="SQL: Execute") -> ("State with Arguments"=w290:string)  [unwired: 4 in]
            n103 = call <vilib>:"Add State(s) to Queue__jki_lib_state_machine.vi"("State(s) in Front (\"\")"=w290, "State(s) in (\"\")"=w297) -> ("States Out"=w296:string)  [unwired: 13 in]
          }
          frame "SQL: Grant Select" {
            # "Your code here.\n(You can make a copy of, or modify, this frame)"
            n104 = Unbundle By Name(w301) -> ()  [unwired: 1 out]
            n105 = call <vilib>:"Build State String with Arguments__JKI_lib_State_Machine.vi"("Arguments (\"\")"="GRANT SELECT ON ALL TABLES IN SCHEMA PUBLIC TO reader;\nGRANT SELECT ON ALL TABLES IN SCHEMA PUBLIC TO llab_reader;" ("format string"), "State"="SQL: Execute") -> ("State with Arguments"=w299:string)  [unwired: 4 in]
            n106 = call <vilib>:"Add State(s) to Queue__jki_lib_state_machine.vi"("State(s) in Front (\"\")"=w299, "State(s) in (\"\")"=w304) -> ("States Out"=w303:string)  [unwired: 13 in]
          }
          frame "SQL: Execute" {
            # "Template Separator\n(You can make a copy of, or modify, this frame)"
            n107 = Unbundle By Name(w305) -> ("LV-Data.PGSQL out"=w311:refnum<class "LV-Data.PGSQL.lvclass">)
            n108 = call "Execute SQL.vi"("error in"=w309, "SQL"=w308, "LV-Data.PGSQL"=w311) -> ("error out"=w310:errorcluster, "LV-Data.PGSQL out"=w307:refnum<class "LV-Data.PGSQL.lvclass">)  [unwired: 5 in, 2 out]
            n109 = Bundle By Name(cluster=w305, "LV-Data.PGSQL out"=w307) -> (w306:T3)
            n110 = call <vilib>:"Add State(s) to Queue__jki_lib_state_machine.vi"("State(s) in (\"\")"=w313) -> ("States Out"=w312:string)  [unwired: 14 in]
          }
        }
      }
      n111 = Unbundle By Name(w12) -> ("LV-Data.PGSQL out"=w18:refnum<class "LV-Data.PGSQL.lvclass">)
    }
    frame Error {
      # "v1 database: table_index instead of hypertables"
      n112 = Equal?(x=w316, y=string[] []) -> (x = y?=w322:bool)
      n113 = case shown="False" w322 {
        tunnel: w316 -> [w327 _]
        tunnel: [w324 0] -> w315
        frame False {
          n114 = for {
            tunnel: w327 -> [w329] mode=indexing
            tunnel: [w328] -> w326 mode=indexing
            n115 = Scan From String(format string="llab_%03d", input string=w329) -> (output 1=w328:i32)  [unwired: 3 in, 3 out]
          }
          n116 = Array Max & Min(array=w326) -> (max value=w325:i32)  [unwired: 3 out]
          n117 = Increment(x=w325) -> (x+1=w324:i32)
        }
        frame True {
        }
      }
      n118 = Format Into String(format string="CREATE TABLE llab_%1$03d(\ntime timestamptz\n);\nCREATE TABLE llab_%1$03d_index(\n\"name\" text UNIQUE,\n\"units\" text,\n\"path\" text PRIMARY KEY\n);\nINSERT INTO llab_%1$03d_index VALUES('time','timestamptz','time');\nINSERT INTO table_index VALUES('%2$s','llab_%1$03d', 'llab_%1$03d', 'llab_%1$03d_index');\nSELECT create_hypertable('llab_%1$03d','time');\n--ALTER TABLE llab_%1$03d OWNER TO tables_owner;\n--ALTER TABLE llab_%1$03d_index OWNER TO tables_owner;\nGRANT SELECT ON ALL TABLES IN SCHEMA PUBLIC TO reader;\nGRANT SELECT ON ALL TABLES IN SCHEMA PUBLIC TO llab_reader;", w315, w314) -> (resulting string=w320:string)  [unwired: 2 in, 1 out]
      n119 = call "Execute SQL.vi"("SQL"=w320, "LV-Data.PGSQL"=w317) -> ("error out"=w319:errorcluster, "LV-Data.PGSQL out"=w318:refnum<class "LV-Data.PGSQL.lvclass">)  [unwired: 6 in, 2 out]
    }
  }
  "Data.PGSQL out" <- w9
  "error out" <- w8
